vi "Clear Stream.vi"(8 "error in (no error)":errorcluster, 10 "stream index":i32, 11 "refnum in":refnum<k20>) -> (0 "error out":errorcluster, 3 "refnum out":refnum<k20>)   [LabVIEW 2015, in "niInstr Streaming v1 Host.lvlib"]
doc: "This VI requests that the stream enter the Idle state. <B>The client is still responsible</B> for clearing out samples that may be pending in the transfer (such as abandoned samples in a Host to Target or Target to Host FIFO).\n\n<B>Input Parameters</B>\n\n<B>error in (no error)</B> 'error in' can accept error information wired from VIs previously called. Use this information to decide if any functionality should be bypassed in the event of errors from other VIs.\n\nRight-click the 'error in' control on the front panel and select 'Explain Error' or 'Explain Warning' from the shortcut menu for more information about the error.\n\n<B>stream index</B> Selects which stream index this VI will interface to. This is the index number at the end of the host interface controls (0..7).\n\n<B>refnum in</B> Wire in the session obtained from Open FPGA Reference.\n\n<B>Output Parameters</B>\n\n<B>error out</B> contains error information. This output provides standard error out functionality.\n\n<B>refnum out</B> Copy of refnum in"
uses:
  <instrlib>/_niInstr/Streaming/v1/Host/niInstr Streaming v1 Host.lvlib
  <instrlib>/_niInstr/Streaming/v1/Common/Stream State.ctl
  <instrlib>/_niInstr/Streaming/v1/Common/niInstr Streaming v1 Common.lvlib
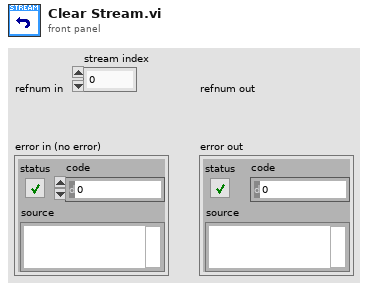
[diagram p1: front panel]
types:
  T1 = typedef "niInstr Streaming v1 Common.lvlib/Stream State.ctl" = enum8{"Idle", "Finite Transfer", "Continuous", "Done", "Error", "Not Ready", "Cancel"}
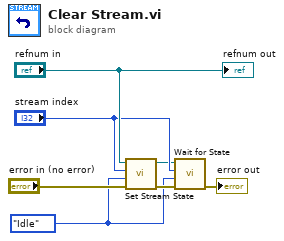
[diagram p0: block diagram]
diagram:
  w1 = Stream_State."Idle" ("Stream State")
  n1 = call <instrlib>:"Set Stream State.vi"("error in (no error)"="error in (no error)", "stream state"=w1, "stream index"="stream index", "refnum in"="refnum in") -> ("error out"=w3:errorcluster, "refnum out"=w2:refnum<k20>)  [unwired: 6 in]
  n2 = call <instrlib>:"Wait for State.vi"("error in (no error)"=w3, "stream state"=w1, "stream index"="stream index", "refnum in"=w2) -> ("error out"=→"error out":errorcluster)  [unwired: 6 in, 1 out]
  "refnum out" <- "refnum in"
